vi "ApplyColorMap.vi"(7 "ColorMap Type":T1, 11 "Image in":u8[][](array[numeric])) -> (3 "Image out":u32[][](array[numeric]))   [LabVIEW 2020]
uses:
  Controls/ColorMap.ctl
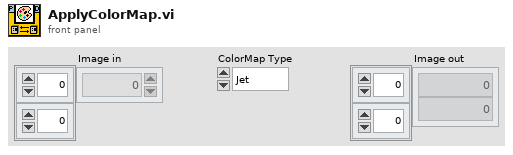
[diagram p1: front panel]
types:
  T1 = typedef "ColorMap.ctl" = enum16{"Jet", "Perula", "Inferno", "Plasma", "Viridis"}
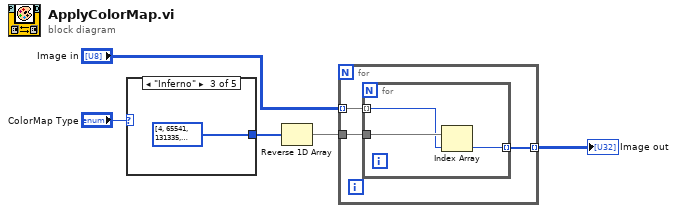
[diagram p0: block diagram]
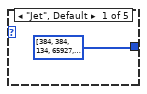
[diagram p2: hidden frame]
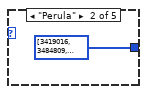
[diagram p3: hidden frame]
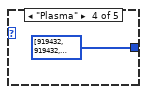
[diagram p4: hidden frame]
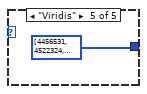
[diagram p5: hidden frame]
diagram:
  n1 = case shown="\"Inferno\"" "ColorMap Type" {
    tunnel: [u32[] [384, 384, 134, 65927, 144, 144, 152, 65689, 160, 65953, 168, 168, 177, 178, 184, 184, 192, 192, 65734, 65734, 208, 208, 65752, 65752, 223, 65760, 232, 489, 241, 498, 248, 66041, 765, 66815, 2558, 134399, 4861, 5375, 6911, 72959, 8958, 75263, 11007, 11263, 13053, 79103, 14845, 146687, 17149, 83455, 19199, 85247, 21502, 22015, 23293, 89599, 25342, 91391, 27390, 158975, 29437, 95743, 31230, 31487, 33277, 165119, 35070, 166655, 37374, 103423, 39421, 171263, 41470, 41983, 43518, 109567, 45308, 177151, 47358, 178943, 49662, 115711, 51454, 183295, 53758, 120063, 55805, 121855, 58367, 58623, 59902, 126207, 61949, 127999, 63999, 195583, 327418, 393211, 786419, 786419, 1310699, 1376236, 1900515, 1900515, 2359260, 2424797, 2949076, 2949076, 3538634, 3604427, 4063171, 4063171, 4521914, 4587451, 4914868, 4980661, 5504939, 5570476, 6028963, 6094756, 6553500, 6619037, 7077523, 7143316, 7732874, 7798667, 8191618, 8257411, 8585081, 8585081, 9043827, 9109364, 9699179, 9699179, 10223203, 10288996, 10747742, 10747742, 11271764, 11337557, 11861836, 11861836, 12255044, 12320581, 12779066, 12844859, 13303605, 13369142, 13827627, 13893420, 14417699, 14483236, 14876189, 14941982, 15466260, 15531797, 16055818, 16121611, 16580101, 16645894, 16775937, 16709888, 16773888, 16642304, 16772097, 16640256, 16769793, 16769536, 16767744, 16636160, 16765697, 16699392, 16763651, 16697601, 16761601, 16630016, 16759553, 16693248, 16757760, 16626176, 16755458, 16689408, 16753411, 16687104, 16751361, 16750592, 16749058, 16748544, 16747010, 16680960, 16745218, 16613376, 16743681, 16677376, 16741376, 16740864, 16739072, 16738560, 16737281, 16736512, 16735490, 16603648, 16733186, 16601600, 16730882, 16730368, 16729090, 16662784, 16727040, 16660992, 16724992, 16658944, 16723202, 16591360, 16720898, 16654848, 16718592, 16652800, 16716802, 16650496, 16714754, 16648704, 16712705, 16646656, 16318721, 16252928, 15925504, 15794176, 15270145, 15204352, 14745857, 14680064, 14156032, 14090240, 13697280, 13631488, 13107715, 13041922, 12648449, 12582912, 12124416, 12058624, 11731200, 11599872, 11075840, 11010048, 10551553, 10485760, 10027010, 9961473, 9502977, 9437184, 8978689, 8847360, 8519680, 8454144] ("jet") u32[] [3419016, 3484809, 3288717, 3288717, 2896532, 2962325, 2766490, 2832283, 2570653, 2636446, 2440356, 2506149, 2048171, 2179757, 1983665, 1983665, 1853367, 1853367, 1591995, 1657788, 1265601, 1265601, 1135302, 1201095, 1005260, 1071053, 809168, 874961, 482776, 548569, 286941, 352734, 287713, 353506, 353760, 419553, 288735, 354528, 355038, 420831, 486876, 486876, 552668, 618461, 684252, 684252, 750299, 816092, 881883, 881883, 816858, 816858, 882902, 948695, 949206, 1014999, 1081047, 1081047, 1146838, 1212631, 1278422, 1278422, 1344468, 1410261, 1344981, 1344981, 1214674, 1280467, 1149649, 1149649, 1084880, 1150673, 1150672, 1150672, 1085649, 1085649, 955342, 955342, 890573, 890573, 890573, 890573, 760267, 826060, 695242, 695242, 630473, 696266, 696265, 762058, 631242, 631242, 435142, 500935, 435910, 435910, 567237, 567237, 698563, 764356, 895423, 961216, 1092541, 1092541, 1354938, 1354938, 1617080, 1682873, 1814197, 1814197, 1880242, 1946035, 2142385, 2208178, 2273711, 2339504, 2536363, 2602156, 2798759, 2864552, 2929830, 2995623, 3258021, 3258021, 3389344, 3455137, 3651999, 3651999, 3848604, 3848604, 4241818, 4307611, 4635287, 4701080, 4962708, 5028501, 5356177, 5421970, 5815183, 5815183, 6142603, 6208396, 6470793, 6536586, 6929542, 6929542, 7191683, 7257476, 7585152, 7650945, 7912830, 7978623, 8371580, 8437373, 8765050, 8765050, 9092726, 9158519, 9420661, 9486454, 9748082, 9879668, 10010225, 10010225, 10403694, 10403694, 10665324, 10731117, 10927467, 10927467, 11189865, 11255658, 11517286, 11517286, 11779428, 11845221, 12041314, 12107107, 12303201, 12368994, 12762465, 12696672, 12958556, 13024349, 13220443, 13286236, 13548123, 13613916, 14007130, 13941337, 14137942, 14203735, 14399829, 14465622, 14531667, 14531667, 14597198, 14662991, 14859852, 14859852, 14991180, 14991180, 15057225, 15057225, 15254085, 15319878, 15319876, 15385669, 15451456, 15451456, 15582781, 15648574, 15910716, 15910716, 15910968, 15976761, 16042550, 16042550, 16239412, 16239412, 16370737, 16436530, 16502063, 16567856, 16502828, 16568621, 16634411, 16700204, 16504104, 16504104, 16504870, 16570663, 16505638, 16505638, 16440867, 16506660, 16506911, 16572704, 16507677, 16507677, 16377373, 16443166, 16443931, 16443931, 16509975, 16575768, 16576277, 16576277, 16445973, 16511766, 16380946, 16380946, 16316175, 16381968, 16448014, 16448014] ("parula") u32[] [4, 65541, 131335, 131335, 65803, 131596, 131598, 131598, 262929, 262929, 328726, 394519, 460061, 525854, 591395, 657188, 788261, 854054, 853801, 919594, 985391, 1051184, 1116723, 1182516, 1313590, 1379383, 1575996, 1641789, 1903683, 1903683, 1969224, 2035017, 2100297, 2166090, 2427982, 2493775, 2689877, 2689877, 2886231, 2952024, 3082842, 3148635, 3410526, 3410526, 3541088, 3606881, 3868772, 3868772, 4065637, 4131430, 4262504, 4262504, 4393577, 4459370, 4656234, 4656234, 4918123, 4983916, 5115243, 5181036, 5312109, 5312109, 5508972, 5574765, 5705838, 5705838, 5902701, 6034287, 6165101, 6230894, 6427502, 6493295, 6559086, 6559086, 6690413, 6756206, 7018351, 7018351, 7149422, 7215215, 7412077, 7477870, 7543404, 7609197, 7806060, 7871853, 8002925, 8068718, 8265068, 8330861, 8462188, 8527981, 8658795, 8724588, 8855915, 8921708, 8987239, 9053032, 9249897, 9315690, 9577833, 9577833, 9708903, 9774696, 9971557, 9971557, 10102884, 10168677, 10365026, 10430819, 10562146, 10627939, 10693730, 10693730, 10956128, 11021921, 11218269, 11284062, 11481181, 11481181, 11546972, 11612765, 11743833, 11809626, 11940950, 12006743, 12072277, 12138070, 12334932, 12400725, 12532050, 12597843, 12728910, 12794703, 12926028, 12991821, 13123149, 13123149, 13320010, 13385803, 13451847, 13517640, 13583431, 13649224, 13780802, 13780802, 13846847, 13978433, 14109502, 14175295, 14241339, 14307132, 14372921, 14438714, 14570039, 14635832, 14701876, 14767669, 14833715, 14899508, 14965551, 15031344, 15097390, 15163183, 15228972, 15294765, 15426604, 15426604, 15492649, 15492649, 15558693, 15624486, 15691041, 15756834, 15822879, 15888672, 15823644, 15889437, 15955482, 16021275, 16087319, 16153112, 16153877, 16219670, 16154642, 16220435, 16221201, 16286994, 16287755, 16353548, 16288522, 16354315, 16420872, 16420872, 16355847, 16487433, 16487942, 16487942, 16554501, 16620294, 16489989, 16555782, 16556296, 16687882, 16557322, 16623115, 16557838, 16689424, 16493585, 16625171, 16494614, 16560407, 16495897, 16561690, 16431132, 16562718, 16497697, 16695076, 16498728, 16564521, 16434220, 16500013, 16369710, 16435503, 16305205, 16370998, 16240442, 16306235, 16175937, 16241730, 16176968, 16242761, 16046923, 16178509, 16047700, 16113493, 16049245, 16115038, 15918434, 16050020, 15788907, 15854700, 15854960, 15986546, 15921531, 15987324, 15856771, 15988357, 15988363, 16119949, 16054675, 16120468, 16251804, 16317597, 16448930, 16580516] ("inferno") u32[] [919432, 919432, 1246857, 1312650, 1705612, 1705612, 1901965, 1967758, 2229903, 2295696, 2491794, 2491794, 2819219, 2885012, 3081621, 3081621, 3212696, 3212696, 3474841, 3474841, 3802266, 3802266, 4064155, 4129948, 4195228, 4261021, 4391839, 4391839, 4588448, 4588448, 4850593, 4916386, 4981409, 5047202, 5243555, 5243555, 5505700, 5505700, 5702052, 5767845, 5833125, 5898918, 6160807, 6160807, 6357159, 6357159, 6488232, 6488232, 6685095, 6685095, 6946984, 6946984, 7078054, 7143591, 7340199, 7405736, 7602599, 7602599, 7733672, 7733672, 7995816, 8061609, 8126889, 8192682, 8389543, 8455336, 8521127, 8521127, 8586662, 8652455, 8849318, 8915111, 9046436, 9112229, 9243300, 9309093, 9375139, 9440932, 9637795, 9703588, 9769378, 9835171, 9966496, 10032289, 10229405, 10295198, 10360987, 10426780, 10492827, 10558620, 10624410, 10690203, 10821783, 10887576, 11018647, 11018647, 11018899, 11150485, 11282324, 11282324, 11348367, 11414160, 11611022, 11676815, 11742606, 11808399, 11939725, 11939725, 12136584, 12202377, 12268424, 12334217, 12400007, 12465800, 12531845, 12597638, 12597889, 12663682, 12729727, 12795520, 12860799, 12992385, 13058430, 13058430, 13124474, 13190267, 13256058, 13321851, 13322104, 13387897, 13453942, 13519735, 13585779, 13651572, 13651568, 13717361, 13914481, 13914481, 13980527, 14046320, 14046571, 14112364, 14178155, 14243948, 14309739, 14375532, 14441577, 14441577, 14507621, 14573414, 14639460, 14639460, 14705505, 14837091, 14837087, 14837087, 14968926, 15034719, 15034717, 15100510, 15101274, 15167067, 15167065, 15232858, 15298904, 15364697, 15430742, 15496535, 15496531, 15562324, 15563090, 15628883, 15694928, 15760721, 15629904, 15695697, 15761740, 15827533, 15893324, 15893324, 15893834, 15959627, 16025672, 16091465, 16026693, 16026693, 16092739, 16158532, 16159043, 16224836, 16290627, 16290627, 16291136, 16356929, 16422975, 16488768, 16423996, 16423996, 16424505, 16490298, 16425273, 16491066, 16426039, 16491832, 16623668, 16623668, 16558387, 16689973, 16559153, 16624946, 16625712, 16691505, 16626478, 16692271, 16692780, 16692780, 16627756, 16693549, 16694060, 16759853, 16564009, 16629802, 16630312, 16696105, 16631078, 16631078, 16566310, 16697896, 16567591, 16567591, 16436773, 16568359, 16568868, 16568868, 16438564, 16504357, 16374052, 16439845, 16375076, 16375076, 16309797, 16375590, 16245285, 16311078, 16181287, 16181287, 15984933, 16116519, 16117032, 16117032, 15986727, 16052520, 15856933, 15856933, 15857443, 15923236] ("plasma") u32[] [4456531, 4522324, 4457560, 4523353, 4523866, 4589659, 4524638, 4590431, 4722017, 4787810, 4657252, 4723045, 4658022, 4723815, 4658791, 4724584, 4594028, 4659821, 4725614, 4791407, 4660591, 4726384, 4661361, 4727154, 4727667, 4859253, 4662903, 4662903, 4729209, 4729209, 4598137, 4729723, 4599420, 4599420, 4599677, 4665470, 4600190, 4665983, 4535680, 4535680, 4470914, 4470914, 4471427, 4471427, 4406148, 4471941, 4472454, 4472454, 4407429, 4407429, 4342662, 4408455, 4212103, 4212103, 4147080, 4212873, 4147337, 4213130, 4082825, 4082825, 3886729, 3952522, 3887499, 3887499, 3756682, 3822475, 3822988, 3822988, 3626636, 3692429, 3692940, 3692940, 3627917, 3627917, 3628428, 3628428, 3498125, 3498125, 3367566, 3367566, 3302284, 3368077, 3237261, 3303054, 3172493, 3238286, 3041934, 3107727, 3107725, 3173518, 3108495, 3108495, 3043213, 3043213, 2912654, 2912654, 2847628, 2913421, 2782349, 2782349, 2782861, 2848654, 2783374, 2783374, 2653069, 2718862, 2653839, 2653839, 2588557, 2588557, 2588814, 2588814, 2523791, 2523791, 2458511, 2524304, 2393486, 2459279, 2393997, 2393997, 2263693, 2329486, 2263950, 2263950, 2133132, 2198925, 2199438, 2199438, 2069131, 2069131, 2069131, 2134924, 2069643, 2069643, 2004620, 2070413, 2005131, 2070924, 1940104, 1940104, 1940615, 2006408, 2072201, 2072201, 2072969, 2072969, 2072965, 2138758, 2204805, 2204805, 2139781, 2139781, 2205574, 2271367, 2337156, 2337156, 2403202, 2468995, 2665858, 2665858, 2797183, 2797183, 2862974, 2928767, 2994811, 3060604, 3191930, 3257723, 3323514, 3323514, 3520375, 3586168, 3717494, 3783287, 3980148, 4045941, 4111474, 4177267, 4439408, 4505201, 4767597, 4833390, 4964715, 5030508, 5161834, 5227627, 5424488, 5490281, 5752423, 5884009, 6080613, 6080613, 6277217, 6343010, 6605664, 6605664, 6868058, 6933851, 7130457, 7196250, 7458645, 7524438, 7852373, 7852373, 8114255, 8180048, 8507983, 8573776, 8639561, 8705354, 8967495, 9033288, 9360964, 9426757, 9819969, 9885762, 10016828, 10148414, 10410554, 10344761, 10738228, 10804021, 11066418, 11132211, 11394094, 11525680, 11722027, 11853613, 12115495, 12115495, 12640295, 12640295, 12771106, 12836899, 13230112, 13295905, 13623581, 13689374, 13885720, 13951513, 14278937, 14344730, 14606873, 14672666, 15000345, 15066138, 15328281, 15394074, 15590427, 15656220, 15918365, 15984158, 16246047, 16377633, 16639524, 16639524] ("viridis")] -> w4
    frame "Jet", Default {
    }
    frame "Perula" {
    }
    frame "Inferno" {
    }
    frame "Plasma" {
    }
    frame "Viridis" {
    }
  }
  n2 = Reverse 1D Array(array=w4) -> (reversed array=w1:u32[])
  n3 = for {
    tunnel: w1 -> [w12]
    tunnel: "Image in" -> [w13] mode=indexing
    tunnel: [w11] -> w2 mode=indexing
    n4 = for {
      tunnel: w13 -> [w15] mode=indexing
      tunnel: w12 -> [w16]
      tunnel: [w14] -> w11 mode=indexing
      n5 = Index Array(array=w16, index=w15) -> (element=w14:u32)
    }
  }
  "Image out" <- w2
